vi "test_AlarmLogic.vi"() -> ()   [LabVIEW 2009]
uses:
  controls/sec_AlarmStates_enum.ctl
  modules/alarms/sec_AlarmLogic_Command_enum.ctl
panel:
  out "Alarm States":T1[](array[typedef])
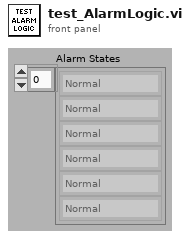
[diagram p1: front panel]
types:
  T1 = typedef "sec_AlarmStates_enum.ctl" = enum16{"Normal", "Alarm", "Bypass", "Tamper"}
  T2 = typedef "sec_AlarmLogic_Command_enum.ctl" = enum16{"Initialise", "Set Alarm Switches", "Check Alarm States", "Get Alarm States"}
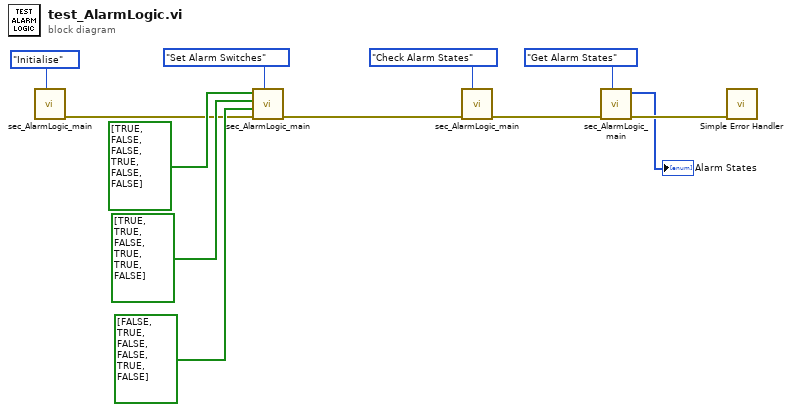
[diagram p0: block diagram]
diagram:
  n1 = call "sec_AlarmLogic_main.vi"("Command"=sec_AlarmLogic_Command_enum."Initialise") -> ("error out"=w3:errorcluster)  [unwired: 9 in, 1 out]
  n2 = call "sec_AlarmLogic_main.vi"("Command"=sec_AlarmLogic_Command_enum."Set Alarm Switches", "error in (no error)"=w3, "Tamper Switches"=bool[] [FALSE, TRUE, FALSE, FALSE, TRUE, FALSE] ("Alarm Switches"), "Bypass Switches"=bool[] [TRUE, TRUE, FALSE, TRUE, TRUE, FALSE] ("Alarm Switches"), "Alarm Switches"=bool[] [TRUE, FALSE, FALSE, TRUE, FALSE, FALSE]) -> ("error out"=w2:errorcluster)  [unwired: 5 in, 1 out]
  n3 = call "sec_AlarmLogic_main.vi"("Command"=sec_AlarmLogic_Command_enum."Check Alarm States", "error in (no error)"=w2) -> ("error out"=w8:errorcluster)  [unwired: 8 in, 1 out]
  n4 = call "sec_AlarmLogic_main.vi"("Command"=sec_AlarmLogic_Command_enum."Get Alarm States", "error in (no error)"=w8) -> ("error out"=w7:errorcluster, "Alarm States"=→"Alarm States":T1[])  [unwired: 8 in]
  n5 = call <vilib>:"Simple Error Handler.vi"("error in (no error)"=w7) -> ()  [unwired: 4 in, 5 out]
